vi "CommIndicator.vi"(6 "Allow":bool, 9 "In3":bool, 10 "In2":bool, 11 "In1":bool) -> (1 "Out3":bool, 2 "Out2":bool, 3 "Out1":bool)   [LabVIEW 2020]
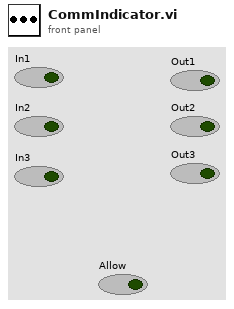
[diagram p1: front panel]
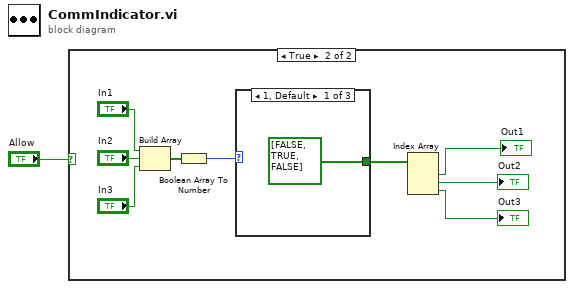
[diagram p0: block diagram]
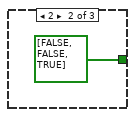
[diagram p3: hidden frame]
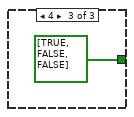
[diagram p4: hidden frame]
diagram:
  n1 = case shown="True" "Allow" {
    frame False {
    }
    frame True {
      n2 = Build Array("In1", "In2", "In3") -> (w7:bool[])
      n3 = Boolean Array To Number(Boolean array=w7) -> (number=w6:u32)
      n4 = case shown="1, Default" w6 {
        tunnel: [bool[] [FALSE, TRUE, FALSE] bool[] [FALSE, FALSE, TRUE] bool[] [TRUE, FALSE, FALSE]] -> w5
        frame 1, Default {
        }
        frame 2 {
        }
        frame 4 {
        }
      }
      n5 = Index Array(array=w5) -> (element #1=→"Out1":bool, element #2=→"Out2":bool, element #3=→"Out3":bool)  [unwired: 3 in]
    }
  }
